vi "Name.CheckSpecialChars.vi"(8 "error in":errorcluster, 11 "Signal Name":string) -> (0 "error out":errorcluster, 3 "Special Character?":bool)   [LabVIEW 2019, in "Diagnostics Addon System Explorer.lvlib"]
uses:
  <vilib>/regexp/Match Regular Expression.xnode
  Diagnostics Addon System Explorer.lvlib
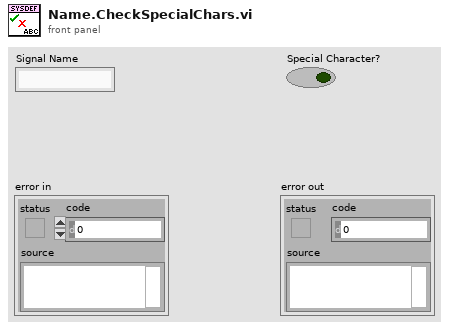
[diagram p1: front panel]
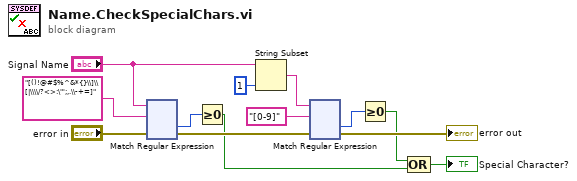
[diagram p0: block diagram]
diagram:
  n1 = xnode "Match Regular Expression"("input string"="Signal Name", "regular expression"="[()!@#$%^&*{}\\]\\[|\\\\/?<>:\"';,.\\-+=]" ("regular expression (\"\")"), "error in"="error in") -> ("offset past match"=w13:i32, "error out"=w8:errorcluster)  [unwired: 3 in, 3 out]
  n2 = Greater Or Equal To 0?(x=w13) -> (x >= 0?=w2:bool)
  n3 = String Subset(string="Signal Name", length (rest)=1 ("length (rest)")) -> (substring=w5:string)  [unwired: 1 in]
  n4 = xnode "Match Regular Expression"("input string"=w5, "regular expression"="[0-9]" ("regular expression (\"\")"), "error in"=w8) -> ("offset past match"=w6:i32, "error out"=→"error out":errorcluster)  [unwired: 3 in, 3 out]
  n5 = Greater Or Equal To 0?(x=w6) -> (x >= 0?=w3:bool)
  n6 = Compound Arithmetic op=OR(w3, w2) -> (→"Special Character?":bool)
